vi "Preliminares.vi"() -> ()   [LabVIEW 2020]
panel:
  out "Waveform Graph":dbl[](graph)
  out "XY Graph":cluster{"X":dbl, "Y":dbl}[](graph)
  out "Frecuencia":ext format="%#.1p"
  out "Operación":string
  out "Pausa [s]":dbl format="%#.1g"
  out "Relación":dbl format="%#.1g"
  out "T_Expiración [s]":dbl format="%#.1g"
  out "FIO2 [%]":u8
  out "Flujo":dbl(graph)
  out "Volúmen":dbl(graph)
  out "Estado":string
  out "T_Inspiración [s]":dbl format="%#.1g"
  out "Presión":dbl(graph)
  in  "Modo":u8(knob) scale=0.0..1.0
  in  "Pausa":sgl(knob) scale=0.0..50.0
  in  "Flujo":dbl(slide) scale=100.0..900.0
  in  "Volúmen":dbl(slide) scale=100.0..800.0
  in  "Estado":u8(knob) scale=0.0..2.0
  in  "FIO2":u8(knob) scale=0.0..13.0
  in  "T_Inspiración":u8(knob) scale=0.0..30.0
  in  "Relación IE":u8(knob) scale=1.0..50.0
  in  "Presión":dbl(slide) scale=50.0..300.0
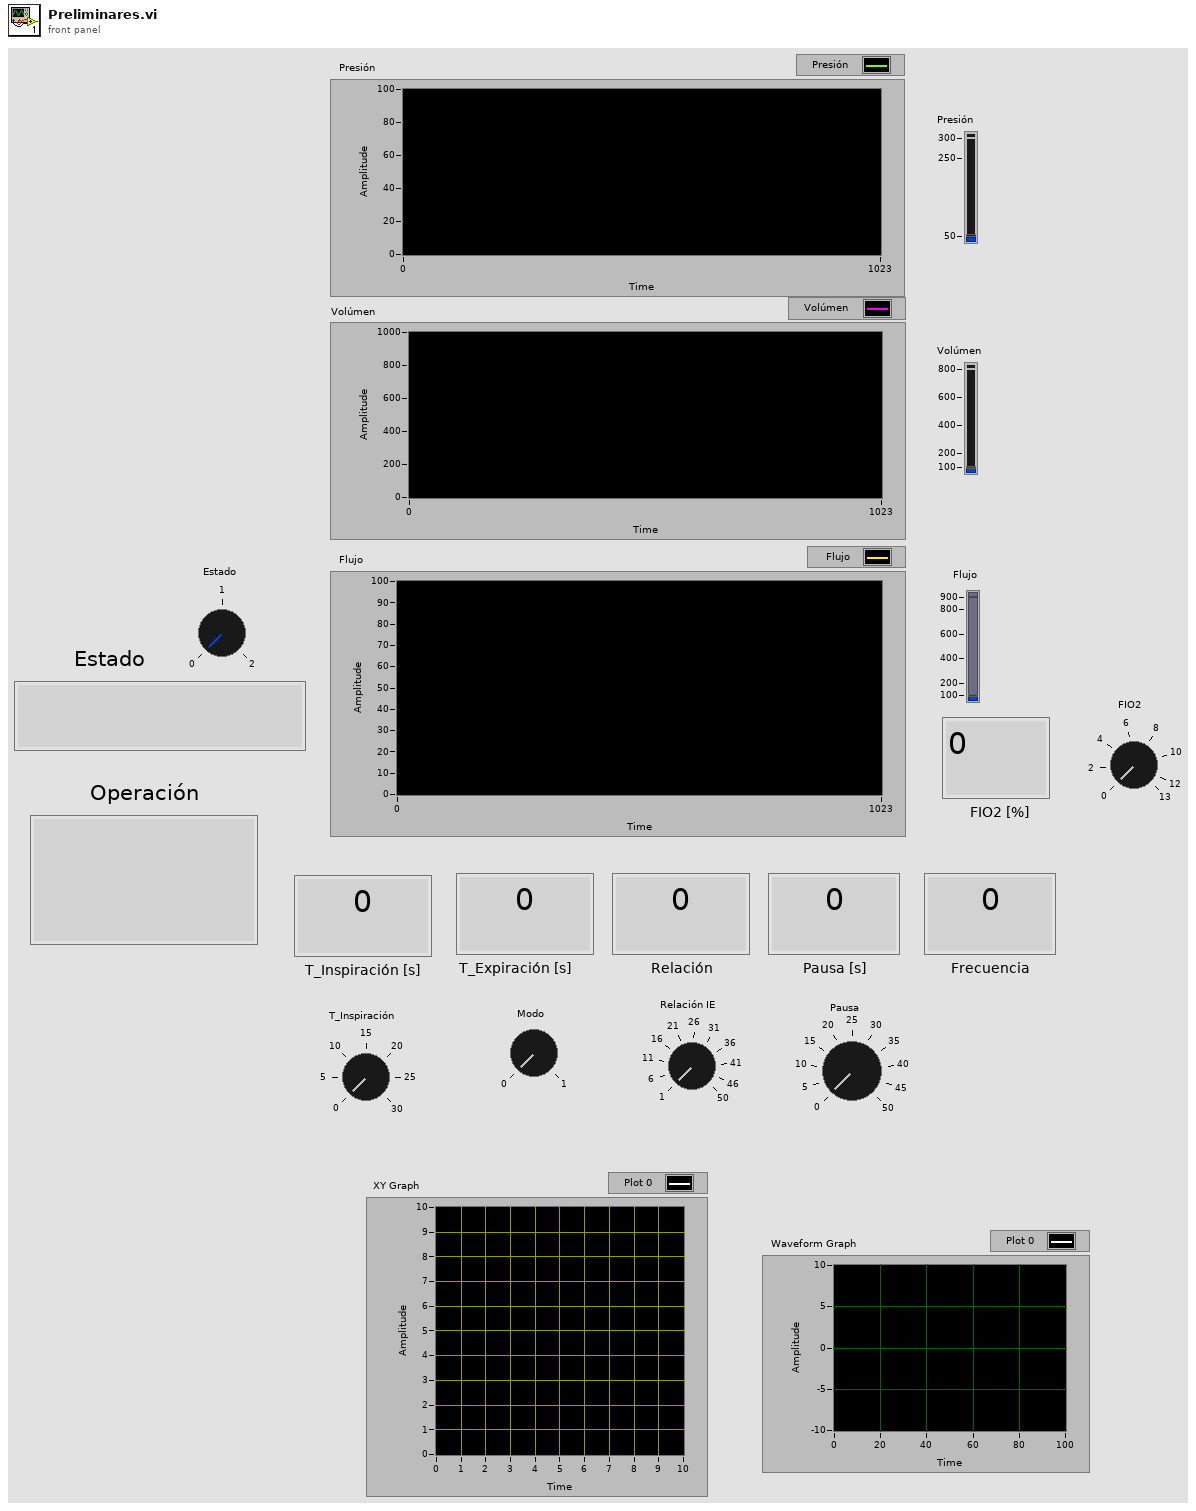
[diagram p1: front panel]
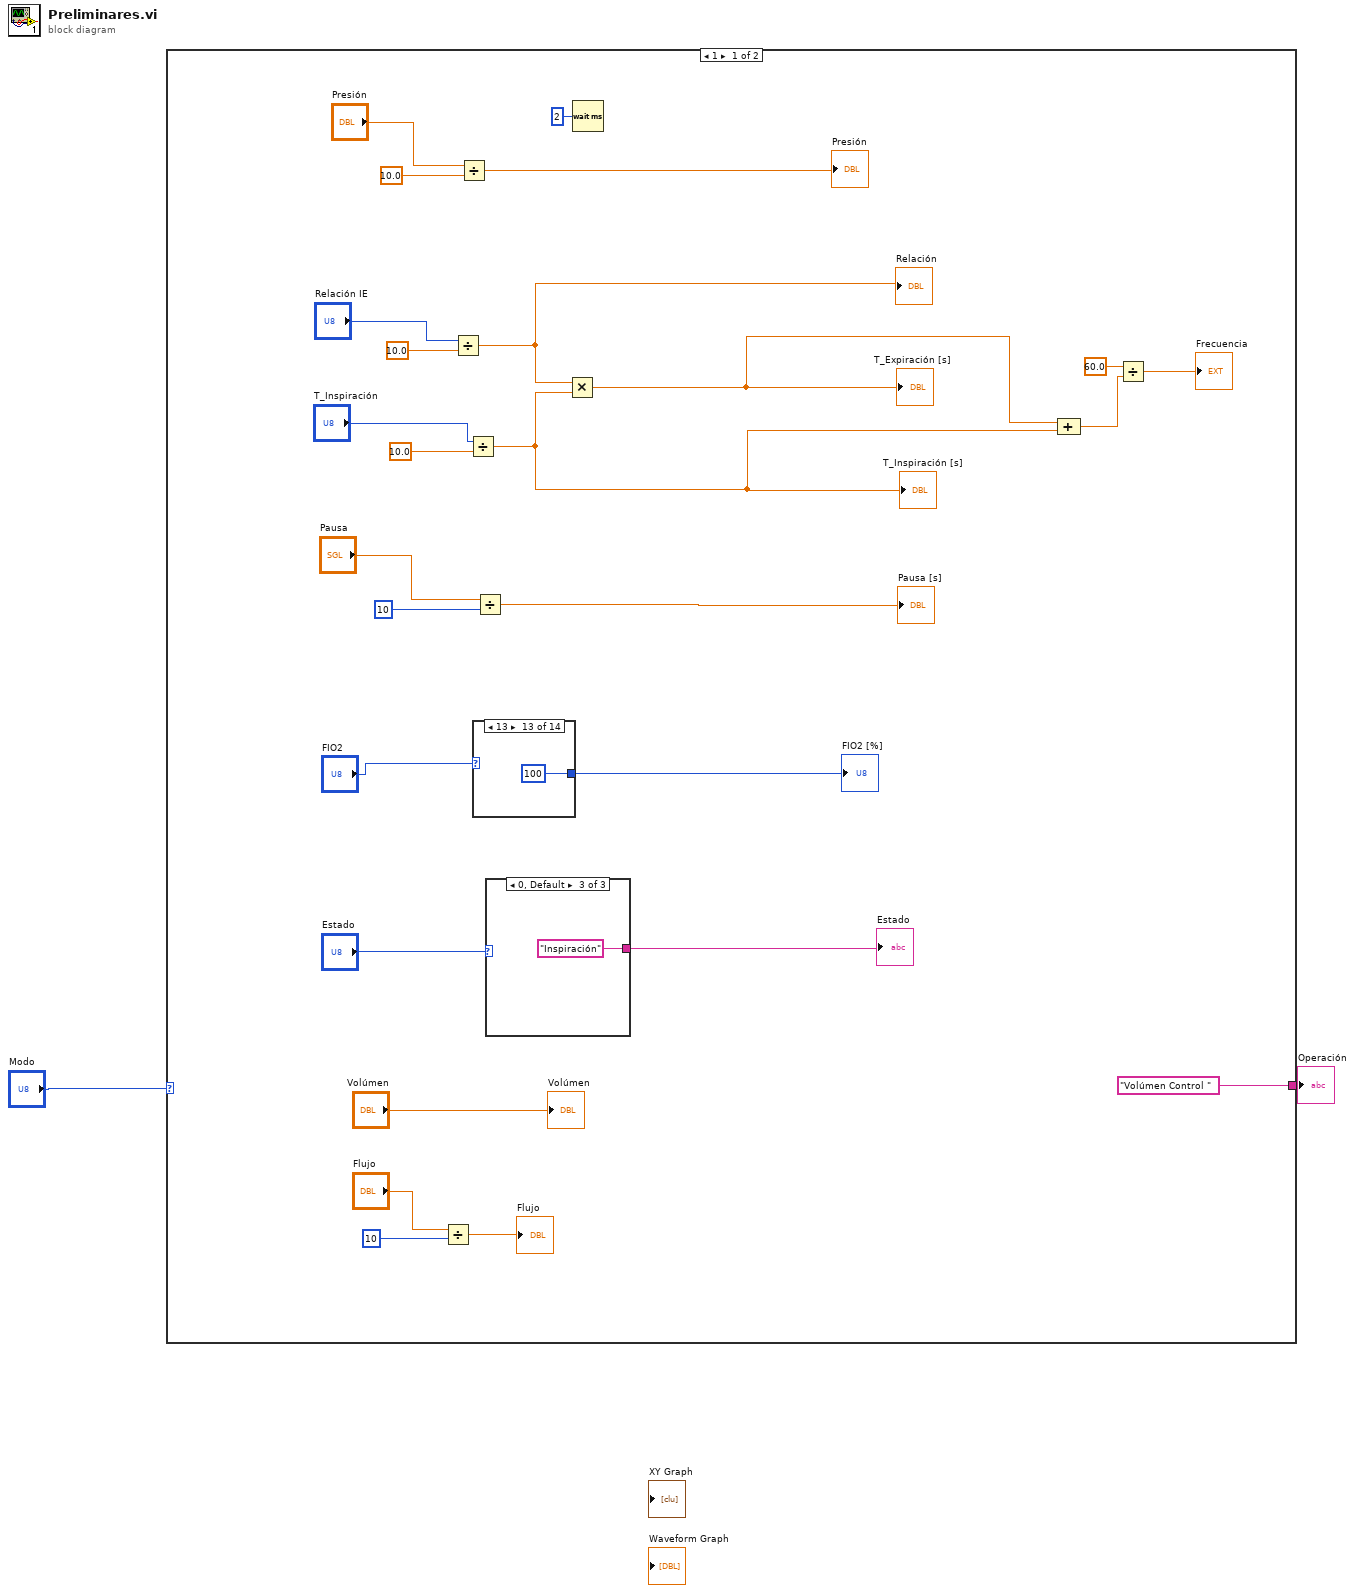
[diagram p0: block diagram]
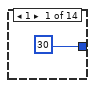
[diagram p2: hidden frame]
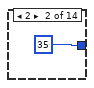
[diagram p3: hidden frame]
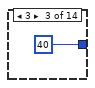
[diagram p4: hidden frame]
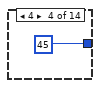
[diagram p5: hidden frame]
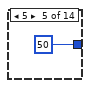
[diagram p6: hidden frame]
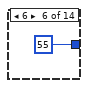
[diagram p7: hidden frame]
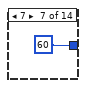
[diagram p8: hidden frame]
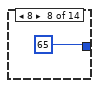
[diagram p9: hidden frame]
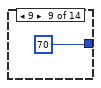
[diagram p10: hidden frame]
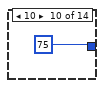
[diagram p11: hidden frame]
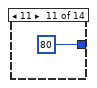
[diagram p12: hidden frame]
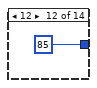
[diagram p13: hidden frame]
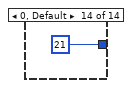
[diagram p14: hidden frame]
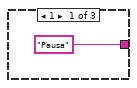
[diagram p15: hidden frame]
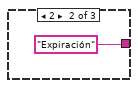
[diagram p16: hidden frame]
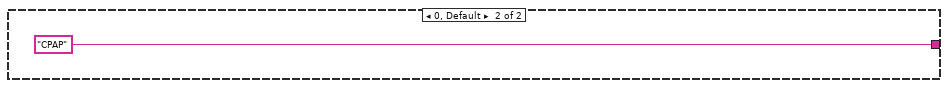
[diagram p17: hidden frame]
diagram:
  n1 = case shown="1" "Modo" {
    tunnel: ["Volúmen Control " "CPAP"] -> w2
    frame 1 {
      n2 = Divide(x="Flujo", y=u8 10) -> (x/y=→"Flujo":dbl)
      n3 = Divide(x="Relación IE", y=10.0) -> (x/y=w14:dbl)
      "Relación" <- w14
      n4 = Divide(x="Presión", y=10.0) -> (x/y=→"Presión":dbl)
      n5 = Divide(x="T_Inspiración", y=10.0) -> (x/y=w8:dbl)
      "T_Inspiración [s]" <- w8
      n6 = case shown="13" "FIO2" {
        tunnel: [30 35 40 45 50 55 60 65 70 75 80 85 100 21] -> w27
        frame 1 {
        }
        frame 2 {
        }
        frame 3 {
        }
        frame 4 {
        }
        frame 5 {
        }
        frame 6 {
        }
        frame 7 {
        }
        frame 8 {
        }
        frame 9 {
        }
        frame 10 {
        }
        frame 11 {
        }
        frame 12 {
        }
        frame 13 {
        }
        frame 0, Default {
        }
      }
      "FIO2 [%]" <- w27
      n7 = Divide(x="Pausa", y=u8 10) -> (x/y=→"Pausa [s]":sgl)
      n8 = case shown="0, Default" "Estado" {
        tunnel: ["Pausa" "Expiración" "Inspiración"] -> w24
        frame 1 {
        }
        frame 2 {
        }
        frame 0, Default {
        }
      }
      "Estado" <- w24
      n9 = Multiply(x=w14, y=w8) -> (x*y=w9:dbl)
      "T_Expiración [s]" <- w9
      n10 = Wait (ms)(milliseconds to wait=u32 2) -> ()  [unwired: 1 out]
      n11 = Compound Arithmetic op=ADD(w9, w8) -> (w11:dbl)
      n12 = Divide(x=60.0, y=w11) -> (x/y=→"Frecuencia":dbl)
      "Volúmen" <- "Volúmen"
    }
    frame 0, Default {
    }
  }
  "Operación" <- w2
